vi "Get Section Name.vi"(8 "error in (no error)":errorcluster, 11 "Configuration File In":refnum<class "Configuration File.lvclass">) -> (0 "error out":errorcluster, 2 "Section Name":string, 3 "Configuration File Out":refnum<class "Configuration File.lvclass">)   [LabVIEW 2020, in "Configuration File.lvclass"]
doc: "Abstract method for reading the assigned name of the object instance. This method must be implemented in the class implementing the interface."
uses:
  Configuration File.lvclass
  Process/Process.lvclass
  Base/Base.lvclass
  Base/Base.lvclass/Base.ctl
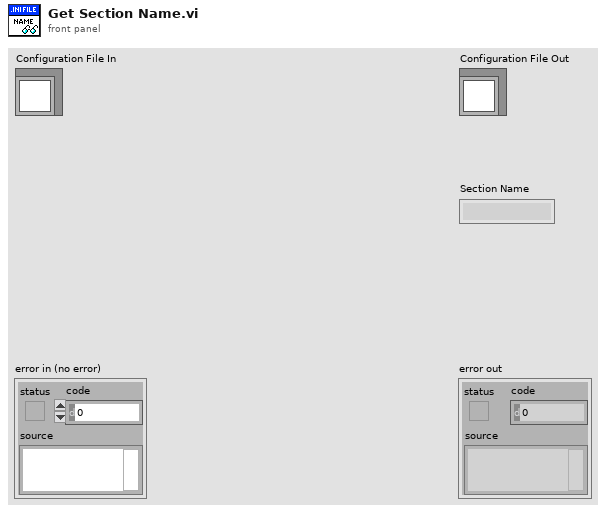
[diagram p1: front panel]
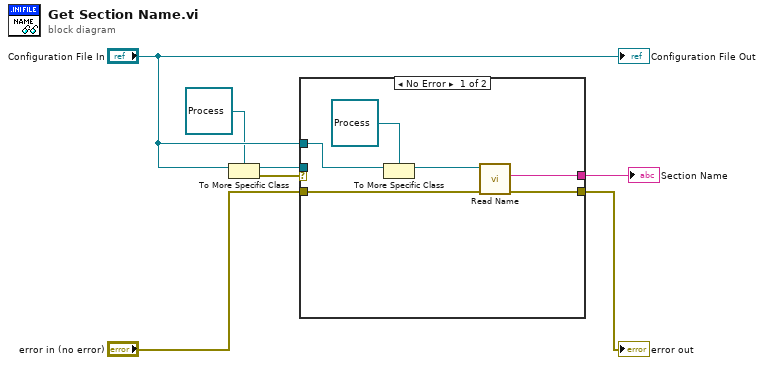
[diagram p0: block diagram]
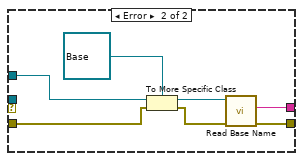
[diagram p2: hidden frame]
diagram:
  n1 = To More Specific Class(target class=refnum<class "Process.lvclass"> refnum ("Process.lvclass"), reference="Configuration File In") -> (specific class reference=w6:refnum<class "Process.lvclass">, error out=w7:errorcluster)  [unwired: 1 in]
  n2 = case shown="No Error" w7 {
    tunnel: w6 -> [_ _]
    tunnel: [w13 w14] -> w5
    tunnel: "Configuration File In" -> [w12 w20]
    tunnel: "error in (no error)" -> [w9 w18]
    tunnel: [w8 w15] -> w1
    frame No Error {
      n3 = To More Specific Class(target class=refnum<class "Process.lvclass"> refnum ("Process.lvclass"), reference=w12) -> (specific class reference=w11:refnum<class "Process.lvclass">)  [unwired: 1 in, 1 out]
      n4 = call "Read Name.vi"("error in (no error)"=w9, "Process In"=w11) -> ("error out"=w8:errorcluster, "Qualified Name"=w13:string)  [unwired: 6 in, 2 out]
    }
    frame Error {
      n5 = To More Specific Class(target class=refnum<class "Base.lvclass"> refnum ("Base.lvclass"), reference=w20, error in=w18) -> (specific class reference=w17:refnum<class "Base.lvclass">, error out=w16:errorcluster)
      n6 = call "Read Base Name.vi"("error in (no error)"=w16, "Base In"=w17) -> ("error out"=w15:errorcluster, "Name"=w14:string)  [unwired: 7 in, 1 out]
    }
  }
  "error out" <- w1
  "Section Name" <- w5
  "Configuration File Out" <- "Configuration File In"
